vi "HW_GEN - Select Used Chan List.vi"(10 "Cfg in":T2[](array[typedef])) -> (1 "VarList":cluster{"Tag":string[], "Alias":string[]}, 2 "UsedChList[]":T1(array[cluster]))   [LabVIEW 2016]
doc: "根据配置信息获取勾选通道的基本信息，包含：\n所属模块的tag，alias\n模块下勾选通道的tag，alias，unit"
uses:
  Ctrls/HardWare _ Module Configuration.ctl
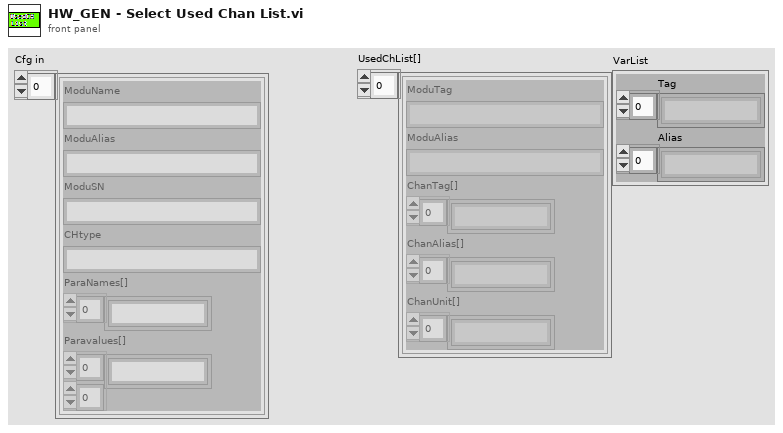
[diagram p1: front panel]
types:
  T1 = cluster{"ModuTag":string, "ModuAlias":string, "ChanTag[]":string[], "ChanAlias[]":string[], "ChanUnit[]":string[]}[]
  T2 = typedef "HardWare _ Module Configuration.ctl" = cluster{"ModuName":string, "ModuAlias":string, "ModuSN":string, "CHtype":string, "ParaNames[]":string[], "Paravalues[]":string[][]}
  T3 = cluster{"ModuTag":string, "ModuAlias":string, "ChanTag[]":string[], "ChanAlias[]":string[], "ChanUnit[]":string[]}
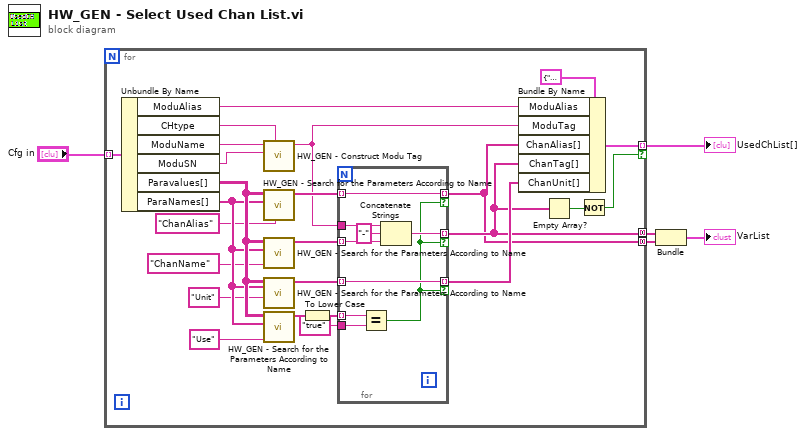
[diagram p0: block diagram]
diagram:
  n1 = for {
    tunnel: "Cfg in" -> [w25] mode=indexing
    tunnel: [w10] -> w4 mode=indexing if=w8
    tunnel: [w7] -> w3 mode=concatenating
    tunnel: [w6] -> w2 mode=concatenating
    n2 = Unbundle By Name(w25) -> ("ModuAlias"=w24:string, "CHtype"=w30:string, "ModuName"=w29:string, "ModuSN"=w28:string, "Paravalues[]"=w27:string[][], "ParaNames[]"=w26:string[])
    n3 = call "HW_GEN - Construct Modu Tag.vi"("ChanType"=w30, "ModSN"=w28, "ModName"=w29) -> ("String"=w13:string)  [unwired: 8 in]
    n4 = call "HW_GEN - Search for the Parameters According to Name.vi"("ParaName"="ChanAlias" ("name"), "ParaNames[]"=w26, "Paravalues[] in"=w27) -> ("Paravalues[] out"=w19:string[])  [unwired: 8 in]
    n5 = call "HW_GEN - Search for the Parameters According to Name.vi"("ParaName"="ChanName" ("name"), "ParaNames[]"=w26, "Paravalues[] in"=w27) -> ("Paravalues[] out"=w18:string[])  [unwired: 8 in]
    n6 = call "HW_GEN - Search for the Parameters According to Name.vi"("ParaName"="Unit" ("name"), "ParaNames[]"=w26, "Paravalues[] in"=w27) -> ("Paravalues[] out"=w17:string[])  [unwired: 8 in]
    n7 = call "HW_GEN - Search for the Parameters According to Name.vi"("ParaName"="Use" ("name"), "ParaNames[]"=w26, "Paravalues[] in"=w27) -> ("Paravalues[] out"=w16:string[])  [unwired: 8 in]
    n8 = To Lower Case(string=w16) -> (all lower case string=w15:string[])
    n9 = for {
      tunnel: w19 -> [w37] mode=indexing
      tunnel: w18 -> [w35] mode=indexing
      tunnel: w17 -> [w32] mode=indexing
      tunnel: w15 -> [w39] mode=indexing
      tunnel: "true" ("name") -> [w38]
      tunnel: [w37] -> w6 mode=indexing if=w31
      tunnel: w13 -> [w36]
      tunnel: [w33] -> w7 mode=indexing if=w31
      tunnel: [w32] -> w11 mode=indexing if=w31
      n10 = Equal?(x=w39, y=w38) -> (x = y?=w31:bool)
      n11 = Concatenate Strings(w36, "-" ("string"), w35) -> (w33:string)
    }
    n12 = Bundle By Name(cluster=T3 {"ModuTag"="", "ModuAlias"="", "ChanTag[]"=[], "ChanAlias[]"=[], "ChanUnit[]"=[]} ("ModuCfg"), "ModuAlias"=w24, "ModuTag"=w13, "ChanAlias[]"=w6, "ChanTag[]"=w7, "ChanUnit[]"=w11) -> (w10:T3)
    n13 = Empty Array?(array=w7) -> (empty?=w9:bool)
    n14 = Not(x=w9) -> (.not. x?=w8:bool)
  }
  "UsedChList[]" <- w4
  n15 = Bundle(w3, w2) -> (→"VarList":cluster{string[], string[]})  [unwired: 1 in]
